vi "Fluke 190 Series II Acquire Scope Measurement.vi"() -> ()   [LabVIEW 2014]
doc: "This example shows how to read a measurement in the scope mode from the instrument."
uses:
  Instance           1 53Saved   Fluke 190 Series II Acquire Scope Measurement .vi
  Public/Data/Read Measurement (Scope Mode).vi
  Fluke 190 Series II.lvlib
panel:
  out "Measurement Value":dbl format="%#.3e"
  in  "Measurement Type (11: Measurement Reading 1)":i32(ring)=11 items=["Measurement Reading 1"=11, "Measurement Reading 2"=21, "Measurement Reading 3"=31, "Measurement Reading 4"=41, "Cursor 1 Absolute Amplitude Value"=61, "Cursor Delta V"=62, "Cursor 2 Absolute Amplitude Value"=71, "Cursor Delta T"=72, "Cursor Maximum"=73, "Cursor Average"=74, "Cursor Minimum"=75, "Cursors Frequency"=76]
  in  "VISA resource name":refnum<visa-resource-name>
  # "(c) 2013-2014 National Instruments.  ALL RIGHTS RESERVED."
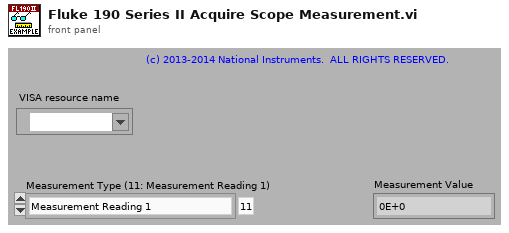
[diagram p1: front panel]
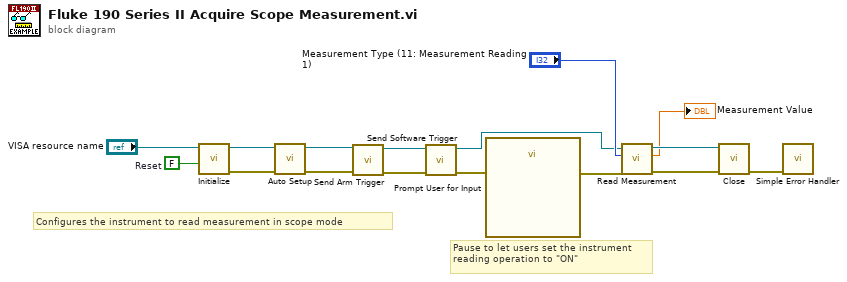
[diagram p0: block diagram]
diagram:
  w15 = FALSE  # Reset
  # "Pause to let users set the instrument\nreading operation to \"ON\""
  # "Configures the instrument to read measurement in scope mode"
  n1 = call "Initialize.vi"("Reset (True)"=w15, "VISA resource name"="VISA resource name") -> ("error out"=w13:errorcluster, "VISA resource name out"=w14:refnum<visa-resource-name>)  [unwired: 2 in, 6 out]
  n2 = call "Auto Setup.vi"("error in (no error)"=w13, "VISA resource name"=w14) -> ("error out"=w11:errorcluster, "VISA resource name out"=w12:refnum<visa-resource-name>)  [unwired: 8 out]
  n3 = call "Send Arm Trigger.vi"("error in (no error)"=w11, "VISA resource name"=w12) -> ("error out"=w9:errorcluster, "VISA resource name out"=w10:refnum<visa-resource-name>)  [unwired: 8 out]
  n4 = call "Send Software Trigger.vi"("error in (no error)"=w9, "VISA resource name"=w10) -> ("error out"=w3:errorcluster, "VISA resource name out"=w1:refnum<visa-resource-name>)  [unwired: 8 out]
  n5 = call "Prompt User for Input"("error in (no error)"=w3) -> ("error out"=w2:errorcluster)  [unwired: 1 in, 17 out]
  n6 = call-poly "Read Measurement.vi"("error in (no error)"=w2, "Measurement Type (11: Measurement Reading 1)"="Measurement Type (11: Measurement Reading 1)", "VISA resource name"=w1) -> ("error out"=w6:errorcluster, "Measurement Value"=→"Measurement Value":dbl, "VISA resource name out"=w7:refnum<visa-resource-name>)  [unwired: 6 out]
  n7 = call "Close.vi"("error in (no error)"=w6, "VISA resource name"=w7) -> ("error out"=w5:errorcluster)  [unwired: 9 out]
  n8 = call <vilib>:"Simple Error Handler.vi"("error in (no error)"=w5) -> ()  [unwired: 1 in, 8 out]
